vi "Dequeue.vi"(8 "error in (no error)":errorcluster, 9 "timeout in ms (-1)":i32=-1, 11 "Message Dequeuer in":refnum<class "Message Dequeuer.lvclass">) -> (0 "error out":errorcluster, 1 "timed out?":bool, 2 "Message":refnum<class "Message.lvclass">, 3 "Message Dequeuer out":refnum<class "Message Dequeuer.lvclass">, 4 "priority":T1=enum."Normal")   [LabVIEW 2020, in "Actor Framework.lvlib" / "Message Dequeuer.lvclass"]
doc: "<p>(<strong>Filename</strong>: <span class=\"dnl\">Actor Framework.lvlib:Message Dequeuer.lvclass:Dequeue.vi</span>)</p>\n\n<p>Reads a message that a top-level actor sent to its caller. Use this VI to interact with non-actor code, not in a VI that belongs to an actor.</p>"
uses:
  Message Dequeuer.lvclass
  Message/Message.lvclass
  Message Dequeuer.lvclass/Message Dequeuer.ctl
  Message Priority Queue/Message Priority Queue.lvclass
  Dequeue Priority.ctl
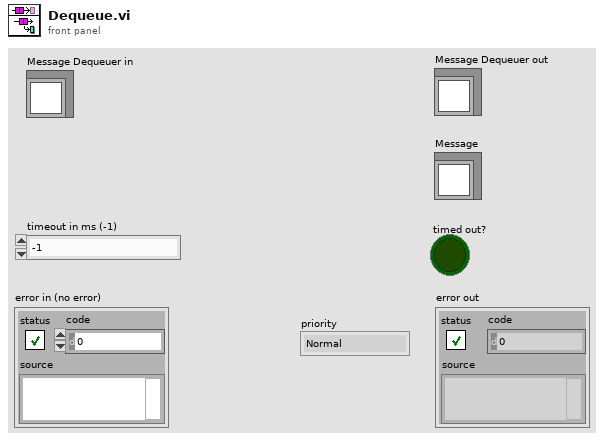
[diagram p1: front panel]
types:
  T1 = typedef "Actor Framework.lvlib/Message Dequeuer.lvclass/Dequeue Priority.ctl" = enum16{"Low", "Normal", "High", "Critical"}
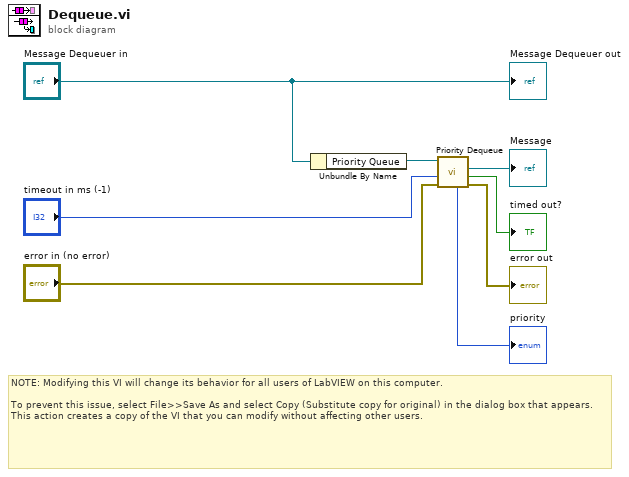
[diagram p0: block diagram]
diagram:
  # "NOTE: Modifying this VI will change its behavior for all users of LabVIEW on this computer.\n\nTo prevent this issue, select File>>Save As and select Copy (Substitute copy for original) in the dialog box that appears. This action creates a copy of the VI that you can modify without affecting other users."
  n1 = Unbundle By Name("Message Dequeuer in") -> ("Priority Queue"=w7:refnum<class "Message Priority Queue.lvclass">)
  n2 = call "Priority Dequeue.vi"("error in (no error)"="error in (no error)", "timeout in ms (-1)"="timeout in ms (-1)", "Priority Queue in"=w7) -> ("error out"=→"error out":errorcluster, "timed out?"=→"timed out?":bool, "element"=→"Message":refnum<class "Message.lvclass">, "priority"=→"priority":i32)  [unwired: 4 in, 1 out]
  "Message Dequeuer out" <- "Message Dequeuer in"
